vi "Copying_day_files.vi"(5 "End time":timestamp, 6 "Start time":timestamp) -> ()   [LabVIEW 2010]
uses:
  Globals/Constants_global.vi
panel:
  out "error out":errorcluster
  out "Path name Out":path
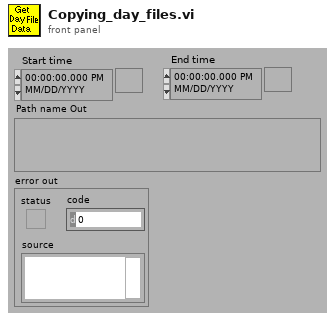
[diagram p1: front panel]
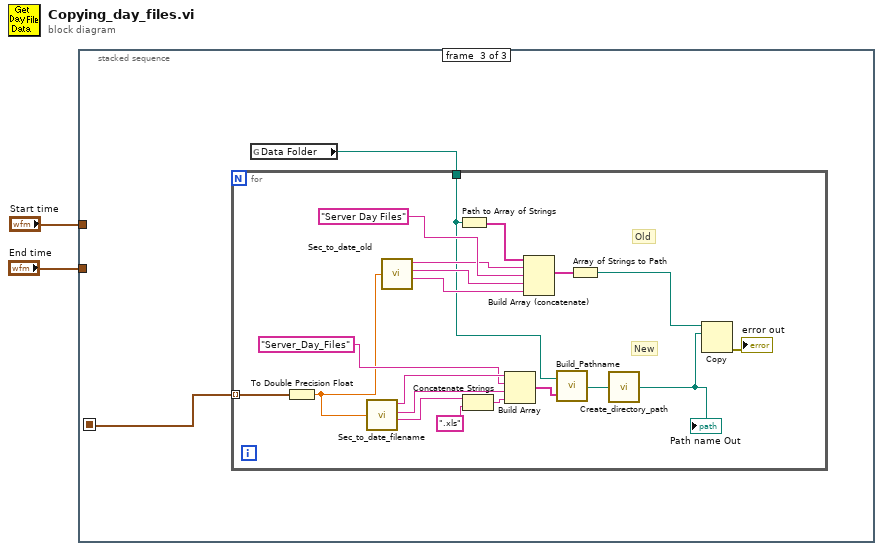
[diagram p0: block diagram]
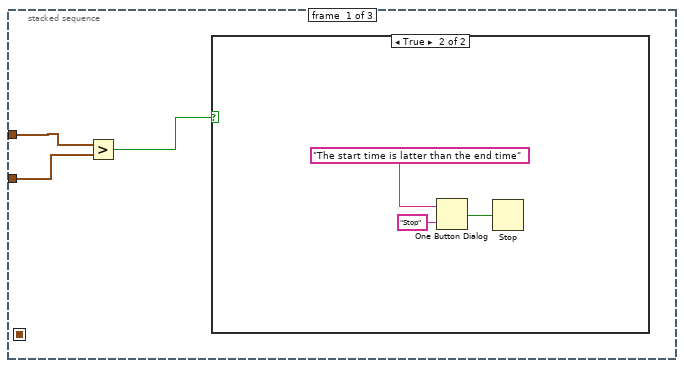
[diagram p2: hidden frame]
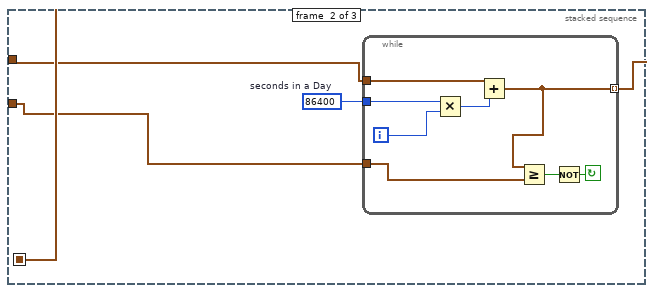
[diagram p4: hidden frame]
diagram:
  n1 = stacked-sequence {
    seq-local: [_ w12 _] -> [_ _ w22]
    tunnel: "End time" -> [w4 w9 _]
    tunnel: "Start time" -> [w3 w10 _]
    frame #0 {
      n2 = Greater?(x=w3, y=w4) -> (0:w5:bool)
      n3 = case shown="True" w5 {
        frame False {
        }
        frame True {
          n4 = One Button Dialog(message="The start time is latter than the end time", button name ("OK")="Stop") -> (true=w7:bool)
          n5 = Stop(stop? (T)=w7) -> ()
        }
      }
    }
    frame #1 {
      w11 = u32 86400  # seconds in a Day
      n6 = while {
        tunnel: [w13] -> w12 mode=indexing
        tunnel: w9 -> [w20]
        tunnel: w10 -> [w14]
        tunnel: w11 -> [w16]
        i -> [w17]
        stop <- w18 continue-if-true
        n7 = Multiply(x=w16, y=w17) -> (x*y=w15:u32)
        n8 = Add(x=w14, y=w15) -> (x+y=w13:timestamp)
        n9 = Greater Or Equal?(x=w13, y=w20) -> (x >= y?=w19:bool)
        n10 = Not(x=w19) -> (.not. x?=w18:bool)
      }
    }
    frame #2 {
      n11 = global read "Constants_global.vi" "Data Folder"() -> (w21:path)
      n12 = for {
        tunnel: w22 -> [w42] mode=indexing
        tunnel: w21 -> [w28]
        # "New"
        # "Old"
        n13 = To Double Precision Float(number=w42) -> (double precision float=w27:dbl)
        n14 = call "Sec_to_date_filename.vi"("seconds"=w27) -> ("Year"=w38:string, "Month"=w37:string, "Day"=w41:string)  [unwired: 1 out]
        n15 = call "Sec_to_date_old.vi"("seconds"=w27) -> ("Year"=w33:string, "Month"=w30:string, "Day"=w31:string)  [unwired: 1 out]
        n16 = Path to Array of Strings(0:w28) -> (2:w29:string[])  [unwired: 1 out]
        n17 = Concatenate Strings(w41, ".xls" ("string")) -> (w39:string)
        n18 = Build Array(w38, "Server_Day_Files" ("Input Element"), w37, w39) -> (w35:string[])
        n19 = Build Array (concatenate)(w29, w33, "Server Day Files" ("Input Element"), w30, w31) -> (w32:string[])
        n20 = call "Build_Pathname.vi"("Output Array"=w35, "Pathname"=w28) -> ("Appended path"=w25:path)
        n21 = Array of Strings to Path(0:w32) -> (2:w26:path)  [unwired: 1 in]
        n22 = call "Create_directory_path.vi"("Path name"=w25) -> ("Path name Out"=w24:path)
        "Path name Out" <- w24
        n23 = Copy(10:w24, 11:w26) -> (0:→"error out":errorcluster)  [unwired: 3 in, 2 out]
      }
    }
  }
